vi "LVClass_HasoData Get HasoSlopes.vi"(0 "HasoData in":refnum<class "HasoData.lvclass">, 5 "HasoSlopes":refnum<class "HasoSlopes.lvclass">, 7 "HasoSlopes raw":refnum<class "HasoSlopes.lvclass">, 11 "error in (no error)":errorcluster) -> (4 "HasoData out":refnum<class "HasoData.lvclass">, 6 "HasoSlopes.dup":refnum<class "HasoSlopes.lvclass">, 8 "HasoSlopes raw":refnum<class "HasoSlopes.lvclass">, 15 "error out":errorcluster)   [LabVIEW 2020, in "HasoData.lvclass"]
doc: "Get raw and processed HasoSlopes objects.\n\n--------------------------------------------------------------------------------\n\n<B>HasoDataIn </B> : HasoData object.\n<B>HasoDataOut </B> : HasoData object.\n<B>HasoSlopes </B> : processed HasoSlopes object.\n<B>HasoSlopesRaw </B> : raw HasoSlopes object.\n<B>ErrorIn </B> : Error\n<B>ErrorOut </B> : Error\n\n--------------------------------------------------------------------------------"
uses:
  HasoData.lvclass
  HasoSlopes.lvclass
  HasoData.lvclass/HasoData.ctl
  LVClass_HasoSlopes Read HasoSlopes _ property.vi
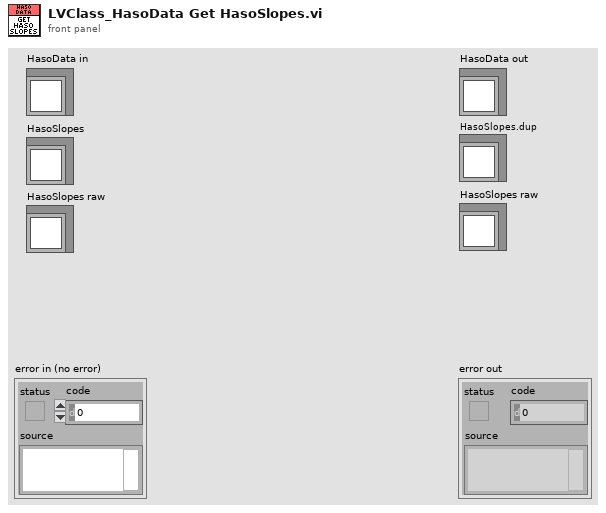
[diagram p1: front panel]
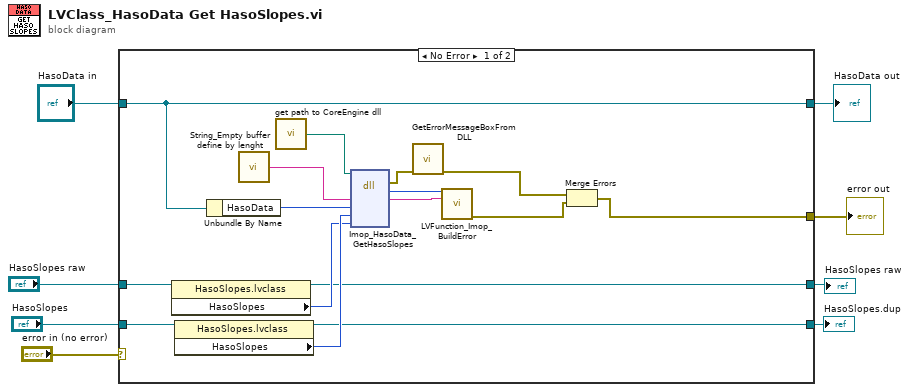
[diagram p0: block diagram]
diagram:
  n1 = case shown="No Error" "error in (no error)" {
    selector: "error in (no error)" -> [_ w27]
    tunnel: [w9 w27] -> w6
    tunnel: [w12 w26] -> w5
    tunnel: "HasoData in" -> [w12 w26]
    tunnel: [w17 w24] -> w4
    tunnel: "HasoSlopes" -> [w17 w24]
    tunnel: "HasoSlopes raw" -> [w16 w25]
    tunnel: [w14 w25] -> w1
    frame No Error {
      n2 = property class="HasoSlopes.lvclass"(reference=w16) -> (reference out=w14:refnum<class "HasoSlopes.lvclass">, "HasoSlopes"=w15:i32)  [unwired: 1 in, 1 out]
      n3 = property class="HasoSlopes.lvclass"(reference=w17) -> ("HasoSlopes"=w18:i32)  [unwired: 1 in, 2 out]
      n4 = Unbundle By Name(w12) -> ("HasoData"=w13:i32)
      n5 = call "String_Empty buffer define by lenght.vi"() -> ("Empty buffer"=w21:string)  [unwired: 1 in]
      n6 = call "get path to CoreEngine dll.vi"() -> ("path to c_interface_vc100.dll"=w20:path)  [unwired: 12 in, 3 out]
      n7 = dll-call lib="D:/2_trunk/temp_core_engine/DLLs/ImopEngine4_vc100.dll" fn="Imop_HasoData_GetHasoSlopes"(path in=w20, "message"=w21, "objet"=w13, "haso slopes"=w18, "HasoSlopesRaw"=w15) -> (error out=w19:errorcluster, "return type"=w23:i32, "message"=w22:string)  [unwired: 5 in, 1 out]
      n8 = call "GetErrorMessageBoxFromDLL.vi"("error IN"=w19) -> ("error OUT"=w11:errorcluster)  [unwired: 10 in]
      n9 = call "LVFunction_Imop_BuildError.vi"("code"=w23, "String to Prepend to source (\"\")"=w22) -> ("error out"=w10:errorcluster)  [unwired: 13 in]
      n10 = Merge Errors(w11, w10) -> (w9:errorcluster)
    }
    frame Error {
    }
  }
  "error out" <- w6
  "HasoData out" <- w5
  "HasoSlopes.dup" <- w4
  "HasoSlopes raw" <- w1
